vi "Read Configuration File.vi"(8 "error in (no error)":errorcluster, 11 "Filepath":path=path "C:/PAS Calibration/Configuration/userConfig.txt") -> (0 "error out":errorcluster, 3 "User Config":T1={"Password"="admin", "cDAQ Name"="cDAQ9188-1A2B7A8", "CAN Interface"=""})   [LabVIEW 2015]
uses:
  User Configuration.ctl
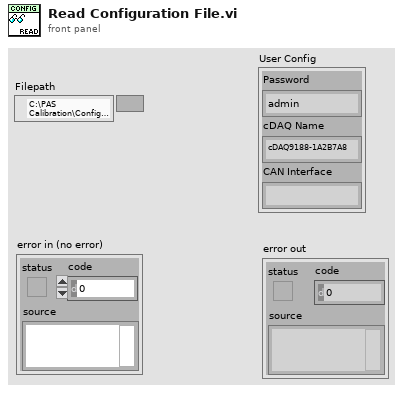
[diagram p1: front panel]
types:
  T1 = typedef "User Configuration.ctl" = cluster{"Password":string, "cDAQ Name":string, "CAN Interface":string}
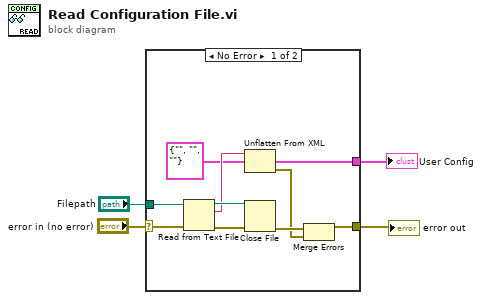
[diagram p0: block diagram]
diagram:
  n1 = case shown="No Error" "error in (no error)" {
    selector: "error in (no error)" -> [w14 w15]
    tunnel: [w8 w15] -> w4
    tunnel: "Filepath" -> [w13 _]
    tunnel: [w6 _] -> w1
    frame No Error {
      n2 = Read from Text File(file (use dialog)=w13, error in=w14) -> (refnum out=w11:refnum<file>, text=w10:string, error out=w12:errorcluster)  [unwired: 2 in, 1 out]
      n3 = Unflatten From XML(xml string=w10, type=T1 {"Password"="", "cDAQ Name"="", "CAN Interface"=""} ("User Config")) -> (value=w6:T1, error out=w7:errorcluster)  [unwired: 1 in]
      n4 = Close File(refnum=w11, error in=w12) -> (error out=w9:errorcluster)  [unwired: 1 out]
      n5 = Merge Errors(w9, w7) -> (w8:errorcluster)
    }
    frame Error {
    }
  }
  "error out" <- w4
  "User Config" <- w1
